vi "rvc Plot 2D Transform (vector).vi"(8 "Error In":errorcluster, 11 "Array of transformations":cluster{"T":dbl[][]}[](array[cluster])) -> (0 "Error Out":errorcluster, 3 "XY Graph":cluster{dbl[], dbl[]}[](graph))   [LabVIEW 2017]
doc: "Given a 3x3 homogenous transformation (T) this function outputs a cluster of the plot components (TrPlot) needed to represent the transformation on an XY Graph."
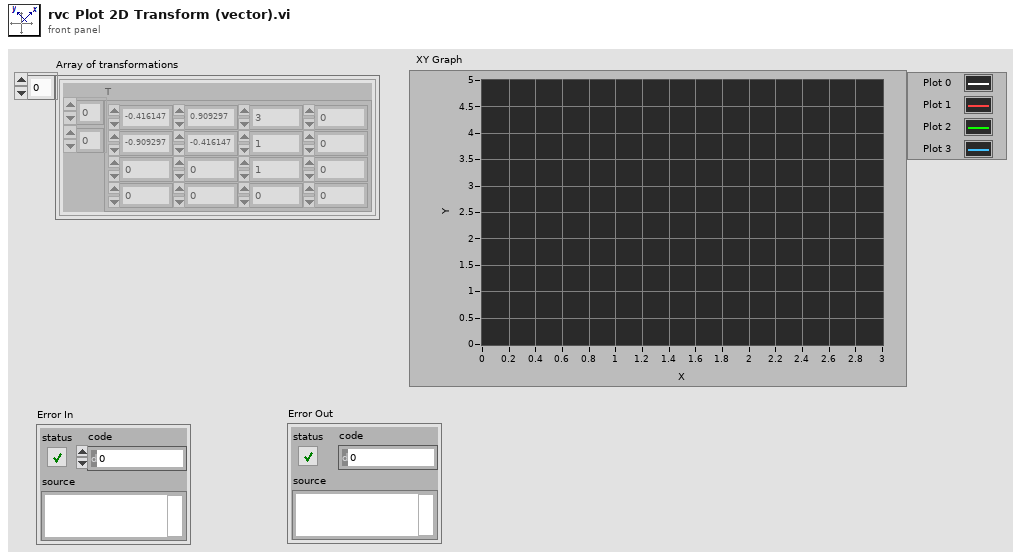
[diagram p1: front panel]
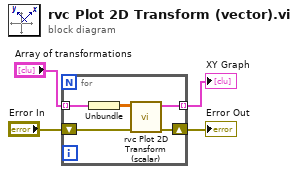
[diagram p0: block diagram]
diagram:
  n1 = for {
    tunnel: [w7] -> w2 mode=indexing
    tunnel: "Array of transformations" -> [w9] mode=indexing
    shift-right: [w5] -> w3
    shift-left: "Error In" -> [w6]
    n2 = Unbundle(w9) -> ("T"=w8:dbl[][])
    n3 = call "rvc Plot 2D Transform (scalar).vi"("Error In"=w6, "T"=w8) -> ("Error Out"=w5:errorcluster, "XY Graph 2"=w7:cluster{dbl[], dbl[]})  [unwired: 8 in]
  }
  "Error Out" <- w3
  "XY Graph" <- w2
